vi "Set Target Velocity MM.vi"(9 "PointStreams":T3, 10 "Input (ft/s)":cluster{"LF":dbl, "LB":dbl, "RF":dbl, "RB":dbl}, 11 "Swerve motors":cluster{"LF":T6, "LB":T6, "RF":T6, "RB":T6}) -> (0 "error out":errorcluster, 3 "PointStreams Out":T2)   [LabVIEW 2020]
uses:
  <vilib>/Rock Robotics/WPI/MotorControl/WPI_MotorControlDeviceRef.ctl
  <vilib>/Rock Robotics/WPI/MotorControl/WPI_MotorControlType.ctl
  <vilib>/Rock Robotics/SystemInterfaces/DIO/FPGA_DIOPWMChannel.ctl
  <vilib>/Rock Robotics/WPI/PWM/WPI_PWMDeadband.ctl
  <vilib>/Rock Robotics/SystemInterfaces/DIO/FPGA_DIOChannel.ctl
  <vilib>/Rock Robotics/WPI/ThirdParty/Phoenix-LabVIEW/Motor Controller/Controls/CTRE_Phoenix_MotorControl_BufferedTrajectoryPointStream_DeviceRef.ctl
  <vilib>/Rock Robotics/WPI/ThirdParty/Phoenix-LabVIEW/Motor Controller/Controls/CTRE_Phoenix_MotorControl_MotionProfileTrajectoryPoint.ctl
  6b64e063-40b4-435e-b595-c1611d5f6bb1.vi
  <vilib>/Rock Robotics/WPI/ThirdParty/Phoenix-LabVIEW/Motor Controller/Get/CTRE_Phoenix_MotorController_GetSelectedSensorData.vi
  Framework/Robot Global Data.vi
  <vilib>/Rock Robotics/WPI/ThirdParty/Phoenix-LabVIEW/Motor Controller/Closed Loop/Motion Profile/CTRE_Phoenix_MotorControl_BufferedTrajectoryPointStream_WriteOne.vi
  <vilib>/ptbypt/NI_PtbyPt.lvlib
panel:
  out "integral x(t) 2":dbl format="%0.2f"
  out "integral x(t)":dbl format="%0.2f"
  in  "Current Pod":T4(ring)
  in  "Push PID":bool
  in  "Debug Mode":bool
  out "Drive Setpoints":T5(graph)
  in  "F":dbl
  in  "D":dbl
  in  "I":dbl
  in  "P":dbl
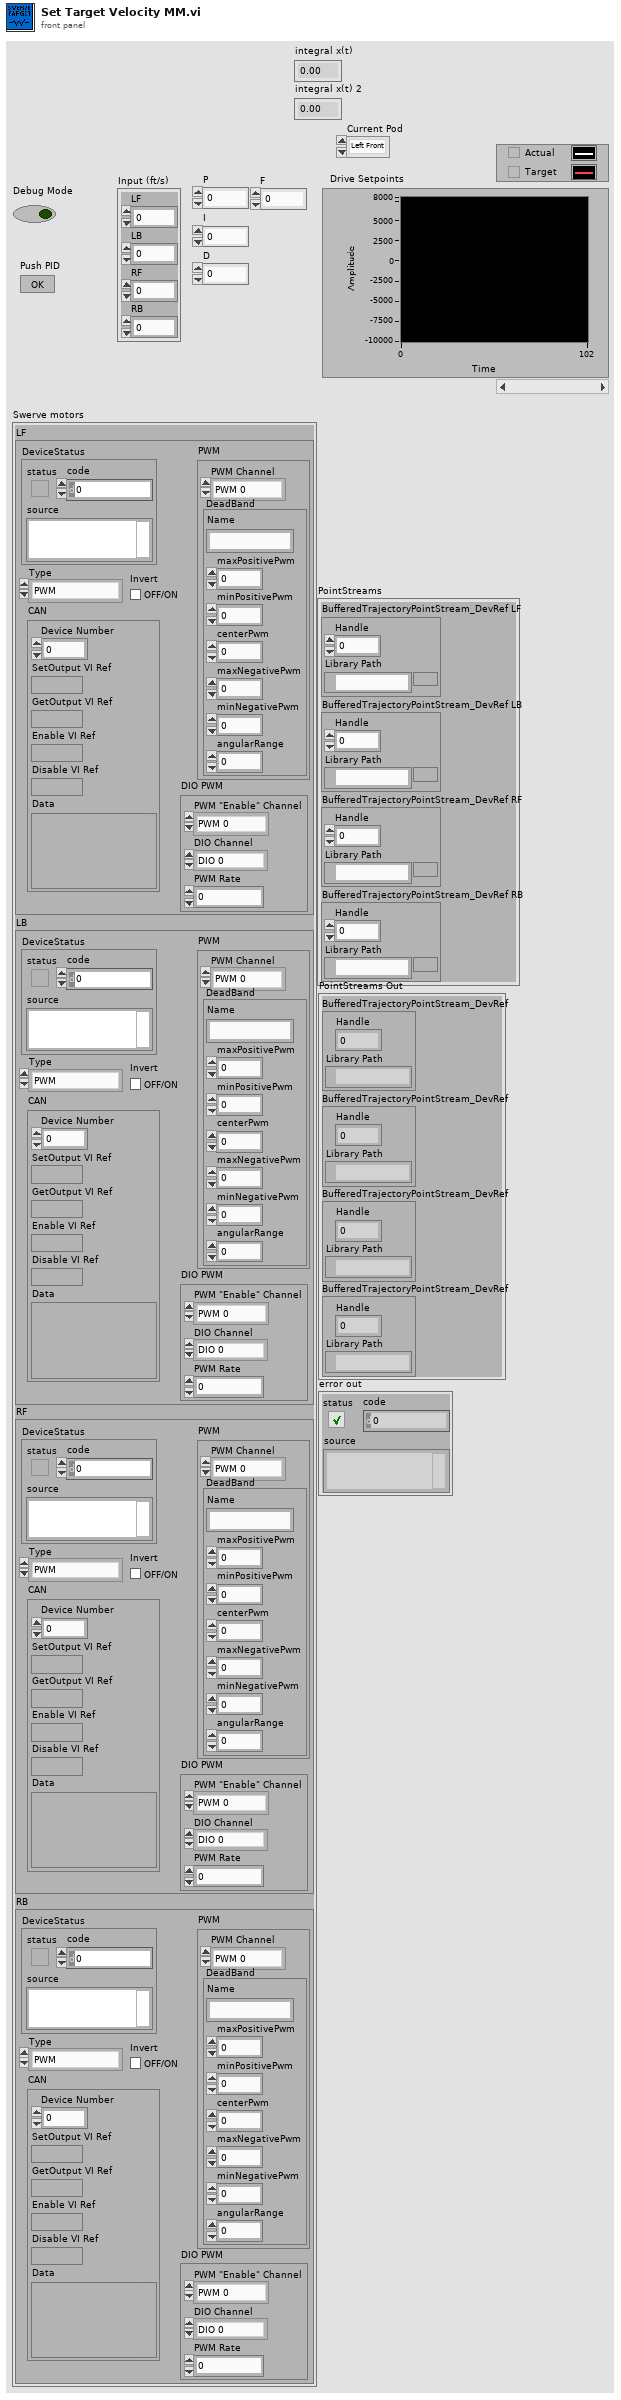
[diagram p1: front panel]
types:
  T1 = typedef "CTRE_Phoenix_MotorControl_BufferedTrajectoryPointStream_DeviceRef.ctl" = cluster{"Handle":u64, "Library Path":path}
  T2 = cluster{"BufferedTrajectoryPointStream_DevRef":T1, "BufferedTrajectoryPointStream_DevRef":T1, "BufferedTrajectoryPointStream_DevRef":T1, "BufferedTrajectoryPointStream_DevRef":T1}
  T3 = cluster{"BufferedTrajectoryPointStream_DevRef LF":T1, "BufferedTrajectoryPointStream_DevRef LB":T1, "BufferedTrajectoryPointStream_DevRef RF":T1, "BufferedTrajectoryPointStream_DevRef RB":T1}
  T4 = enum16{"Left Front", "Left Back", "Right Front", "Right Back"}
  T5 = cluster{"Velocity (Raw Sensor Units per 100 ms)":i32, "Velocity (ticks/ds)":dbl}
  T6 = typedef "WPI_MotorControlDeviceRef.ctl" = cluster{"DeviceStatus":errorcluster, "Type":T7, "PWM":cluster{"PWM Channel":T8, "DeadBand":T9}, "CAN":cluster{"Device Number":u8, "SetOutput VI Ref":variant, "GetOutput VI Ref":variant, "Enable VI Ref":variant, "Disable VI Ref":variant, "Data":variant}, "Invert":bool, "DIO PWM":cluster{"PWM \"Enable\" Channel":T8, "DIOChannel":T10, "PWM Rate":dbl}}
  T7 = typedef "WPI_MotorControlType.ctl" = enum16{"PWM", "CAN", "DIO PWM"}
  T8 = typedef "FPGA_DIOPWMChannel.ctl" = enum8{"PWM 0", "PWM 1", "PWM 2", "PWM 3", "PWM 4", "PWM 5", "PWM 6", "PWM 7", "PWM 8", "PWM 9", "PWM MXP 0", "PWM MXP 1", "PWM MXP 2", "PWM MXP 3", "PWM MXP 4", "PWM MXP 5", "PWM MXP 6", "PWM MXP 7", "PWM MXP 8", "PWM MXP 9", "Invalid"}
  T9 = typedef "WPI_PWMDeadband.ctl" = cluster{"Name":string, "maxPositivePwm":i32, "minPositivePwm":i32, "centerPwm":i32, "maxNegativePwm":i32, "minNegativePwm":i32, "angularRange":u16}
  T10 = typedef "FPGA_DIOChannel.ctl" = enum8{"DIO 0", "DIO 1", "DIO 2", "DIO 3", "DIO 4", "DIO 5", "DIO 6", "DIO 7", "DIO 8", "DIO 9", "DIO MXP 0", "DIO MXP 1", "DIO MXP 2", "DIO MXP 3", "DIO MXP 4", "DIO MXP 5", "DIO MXP 6", "DIO MXP 7", "DIO MXP 8", "DIO MXP 9", "DIO MXP 10", "DIO MXP 11", "DIO MXP 12", "DIO MXP 13", "DIO MXP 14", "DIO MXP 15", "SPI Port CS1", "SPI Port CS2", "SPI Port CS3", "SPI Port MISO", "SPI Port MOSI", "Invalid"}
  T11 = typedef "CTRE_Phoenix_MotorControl_MotionProfileTrajectoryPoint.ctl" = cluster{"Position":dbl, "Velocity":dbl, "Arbitrary Feed Forward":dbl, "Auxiliary Position":dbl, "Auxiliary Velocity":dbl, "Auxiliary Arbitrary Feed Forward":dbl, "Profile Slot Select":i32, "Auxiliary Profile Slot Select":i32, "isLastPoint?":bool, "Zero Position?":bool, "durationMs":u32, "Use Aux PID?":bool}
  T12 = cluster{"LF":bool, "LB":bool, "RF":bool, "RB":bool}
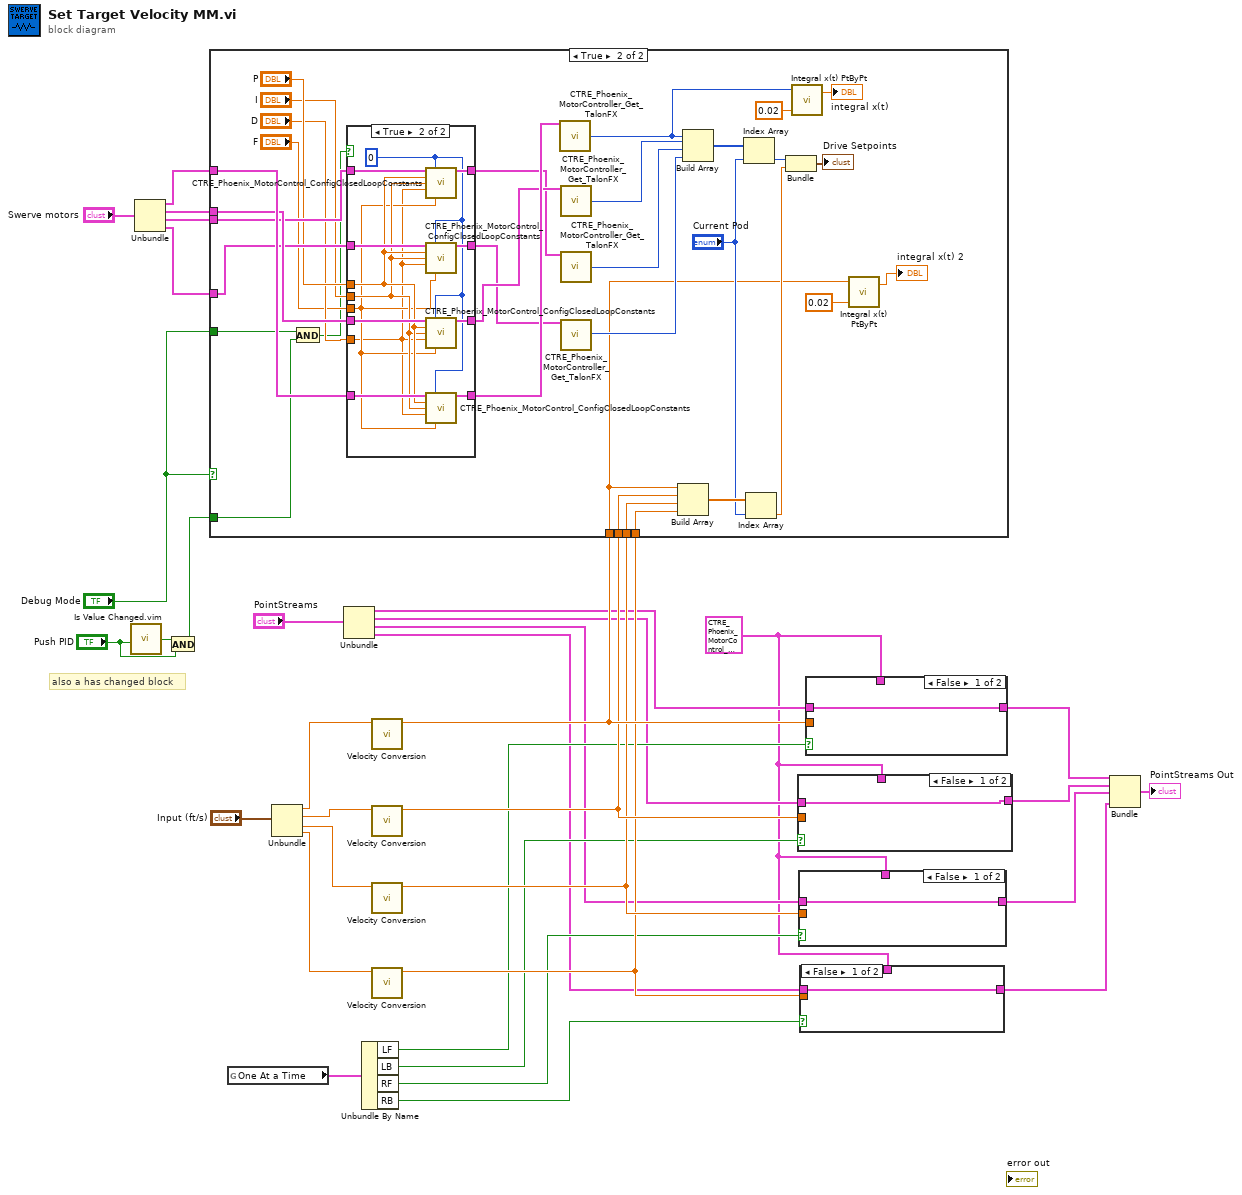
[diagram p0: block diagram]
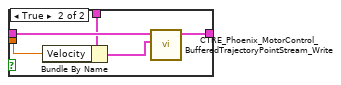
[diagram p2: hidden frame]
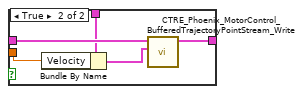
[diagram p3: hidden frame]
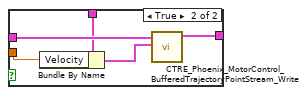
[diagram p4: hidden frame]
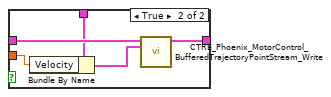
[diagram p5: hidden frame]
diagram:
  w6 = T11 {"Position"=0.0, "Velocity"=0.0, "Arbitrary Feed Forward"=0.0, "Auxiliary Position"=0.0, "Auxiliary Velocity"=0.0, "Auxiliary Arbitrary Feed Forward"=0.0, "Profile Slot Select"=0, "Auxiliary Profile Slot Select"=0, "isLastPoint?"=FALSE, "Zero Position?"=FALSE, "durationMs"=0, "Use Aux PID?"=FALSE} ("element")
  # "also a has changed block"
  n1 = call "Is Value Changed.vim"("value"="Push PID") -> ("changed or first call?"=w18:bool)
  n2 = Unbundle("Swerve motors") -> ("LF"=w33:T6, "LB"=w32:T6, "RF"=w31:T6, "RB"=w30:T6)
  n3 = And(x=w18, y="Push PID") -> (x .and. y?=w19:bool)
  n4 = global read "Robot Global Data.vi" "One At a Time"() -> (w16:T12)
  n5 = Unbundle("Input (ft/s)") -> ("LF"=w28:dbl, "LB"=w27:dbl, "RF"=w26:dbl, "RB"=w25:dbl)
  n6 = Unbundle("PointStreams") -> ("BufferedTrajectoryPointStream_DevRef LF"=w10:T1, "BufferedTrajectoryPointStream_DevRef LB"=w9:T1, "BufferedTrajectoryPointStream_DevRef RF"=w8:T1, "BufferedTrajectoryPointStream_DevRef RB"=w7:T1)
  n7 = Unbundle By Name(w16) -> ("LF"=w15:bool, "LB"=w14:bool, "RF"=w13:bool, "RB"=w12:bool)
  n8 = call "Velocity Conversion.vi"("Velocity (ft/s)"=w28) -> ("Velocity (ticks/ds)"=w24:dbl)  [unwired: 10 in]
  n9 = call "Velocity Conversion.vi"("Velocity (ft/s)"=w27) -> ("Velocity (ticks/ds)"=w23:dbl)  [unwired: 10 in]
  n10 = call "Velocity Conversion.vi"("Velocity (ft/s)"=w26) -> ("Velocity (ticks/ds)"=w22:dbl)  [unwired: 10 in]
  n11 = call "Velocity Conversion.vi"("Velocity (ft/s)"=w25) -> ("Velocity (ticks/ds)"=w21:dbl)  [unwired: 10 in]
  n12 = case shown="True" "Debug Mode" {
    tunnel: w33 -> [_ w67]
    tunnel: w32 -> [_ w66]
    tunnel: w31 -> [_ w65]
    tunnel: w30 -> [_ w64]
    tunnel: w24 -> [_ w36]
    tunnel: w23 -> [_ w49]
    tunnel: w22 -> [_ w48]
    tunnel: w21 -> [_ w47]
    tunnel: "Debug Mode" -> [_ w54]
    tunnel: w19 -> [_ w53]
    frame False {
    }
    frame True {
      n13 = And(x=w54, y=w53) -> (x .and. y?=w55:bool)
      n14 = case shown="True" w55 {
        tunnel: w67 -> [w71 w84]
        tunnel: w66 -> [w70 w83]
        tunnel: w65 -> [w69 w82]
        tunnel: w64 -> [w68 w81]
        tunnel: "P" -> [_ w80]
        tunnel: "I" -> [_ w79]
        tunnel: "D" -> [_ w72]
        tunnel: "F" -> [_ w78]
        tunnel: [w71 w77] -> w59
        tunnel: [w70 w76] -> w58
        tunnel: [w69 w75] -> w57
        tunnel: [w68 w74] -> w56
        frame False {
        }
        frame True {
          w73 = 0 ("slotIdx")
          n15 = call <vilib>:"CTRE_Phoenix_MotorControl_ConfigClosedLoopConstants.vi"("PhoenixMotorControlDevRef"=w82, "slotIdx"=w73, "P"=w80, "I"=w79, "D"=w72, "F"=w78) -> ("PhoenixMotorControlDevRef"=w75:T6)  [unwired: 8 in, 1 out]
          n16 = call <vilib>:"CTRE_Phoenix_MotorControl_ConfigClosedLoopConstants.vi"("PhoenixMotorControlDevRef"=w81, "slotIdx"=w73, "P"=w80, "I"=w79, "D"=w72, "F"=w78) -> ("PhoenixMotorControlDevRef"=w74:T6)  [unwired: 8 in, 1 out]
          n17 = call <vilib>:"CTRE_Phoenix_MotorControl_ConfigClosedLoopConstants.vi"("PhoenixMotorControlDevRef"=w83, "slotIdx"=w73, "P"=w80, "I"=w79, "D"=w72, "F"=w78) -> ("PhoenixMotorControlDevRef"=w76:T6)  [unwired: 8 in, 1 out]
          n18 = call <vilib>:"CTRE_Phoenix_MotorControl_ConfigClosedLoopConstants.vi"("PhoenixMotorControlDevRef"=w84, "slotIdx"=w73, "P"=w80, "I"=w79, "D"=w72, "F"=w78) -> ("PhoenixMotorControlDevRef"=w77:T6)  [unwired: 8 in, 1 out]
        }
      }
      n19 = call-poly <vilib>:"CTRE_Phoenix_MotorController_Get_TalonFX.vi"("PhoenixMotorControlDevRef"=w59) -> ("Velocity (Raw Sensor Units per 100 ms)"=w40:i32)  [unwired: 11 in, 3 out]
      n20 = call-poly <vilib>:"CTRE_Phoenix_MotorController_Get_TalonFX.vi"("PhoenixMotorControlDevRef"=w58) -> ("Velocity (Raw Sensor Units per 100 ms)"=w52:i32)  [unwired: 11 in, 3 out]
      n21 = call-poly <vilib>:"CTRE_Phoenix_MotorController_Get_TalonFX.vi"("PhoenixMotorControlDevRef"=w57) -> ("Velocity (Raw Sensor Units per 100 ms)"=w51:i32)  [unwired: 11 in, 3 out]
      n22 = call-poly <vilib>:"CTRE_Phoenix_MotorController_Get_TalonFX.vi"("PhoenixMotorControlDevRef"=w56) -> ("Velocity (Raw Sensor Units per 100 ms)"=w50:i32)  [unwired: 11 in, 3 out]
      n23 = Build Array(w36, w49, w48, w47) -> (w45:dbl[])
      n24 = Build Array(w40, w52, w51, w50) -> (w46:i32[])
      n25 = Index Array(array=w46, index="Current Pod") -> (element=w43:i32)
      n26 = Index Array(array=w45, index="Current Pod") -> (element=w42:dbl)
      n27 = Bundle("Velocity (Raw Sensor Units per 100 ms)"=w43, "Velocity (ticks/ds)"=w42) -> (→"Drive Setpoints":T5)  [unwired: 1 in]
      n28 = call <vilib>:"Integral x(t) PtByPt.vi"("dt"=0.02, "x"=w40) -> ("integral x(t)"=→"integral x(t)":dbl)  [unwired: 2 in, 1 out]
      n29 = call <vilib>:"Integral x(t) PtByPt.vi"("dt"=0.02, "x"=w36) -> ("integral x(t)"=→"integral x(t) 2":dbl)  [unwired: 2 in, 1 out]
    }
  }
  n30 = case shown="False" w14 {
    tunnel: w23 -> [_ w89]
    tunnel: w9 -> [w85 w90]
    tunnel: w6 -> [_ w87]
    tunnel: [w85 w86] -> w4
    frame False {
    }
    frame True {
      n31 = Bundle By Name(cluster=w87, "Velocity"=w89) -> (w88:T11)
      n32 = call-poly <vilib>:"CTRE_Phoenix_MotorControl_BufferedTrajectoryPointStream_Write.vi"("Trajectory Point"=w88, "BufferedTrajectoryPointStream_DevRef"=w90) -> ("BufferedTrajectoryPointStream_DevRef"=w86:T1)  [unwired: 8 in, 1 out]
    }
  }
  n33 = case shown="False" w13 {
    tunnel: w22 -> [_ w95]
    tunnel: w8 -> [w91 w96]
    tunnel: w6 -> [_ w94]
    tunnel: [w91 w92] -> w3
    frame False {
    }
    frame True {
      n34 = Bundle By Name(cluster=w94, "Velocity"=w95) -> (w93:T11)
      n35 = call-poly <vilib>:"CTRE_Phoenix_MotorControl_BufferedTrajectoryPointStream_Write.vi"("Trajectory Point"=w93, "BufferedTrajectoryPointStream_DevRef"=w96) -> ("BufferedTrajectoryPointStream_DevRef"=w92:T1)  [unwired: 8 in, 1 out]
    }
  }
  n36 = case shown="False" w12 {
    tunnel: w21 -> [_ w101]
    tunnel: w7 -> [w97 w102]
    tunnel: w6 -> [_ w100]
    tunnel: [w97 w98] -> w2
    frame False {
    }
    frame True {
      n37 = Bundle By Name(cluster=w100, "Velocity"=w101) -> (w99:T11)
      n38 = call-poly <vilib>:"CTRE_Phoenix_MotorControl_BufferedTrajectoryPointStream_Write.vi"("Trajectory Point"=w99, "BufferedTrajectoryPointStream_DevRef"=w102) -> ("BufferedTrajectoryPointStream_DevRef"=w98:T1)  [unwired: 8 in, 1 out]
    }
  }
  n39 = case shown="False" w15 {
    tunnel: w24 -> [_ w105]
    tunnel: w10 -> [w103 w108]
    tunnel: w6 -> [_ w107]
    tunnel: [w103 w104] -> w5
    frame False {
    }
    frame True {
      n40 = Bundle By Name(cluster=w107, "Velocity"=w105) -> (w106:T11)
      n41 = call-poly <vilib>:"CTRE_Phoenix_MotorControl_BufferedTrajectoryPointStream_Write.vi"("Trajectory Point"=w106, "BufferedTrajectoryPointStream_DevRef"=w108) -> ("BufferedTrajectoryPointStream_DevRef"=w104:T1)  [unwired: 8 in, 1 out]
    }
  }
  n42 = Bundle("BufferedTrajectoryPointStream_DevRef"=w5, "BufferedTrajectoryPointStream_DevRef"=w4, "BufferedTrajectoryPointStream_DevRef"=w3, "BufferedTrajectoryPointStream_DevRef"=w2) -> (→"PointStreams Out":T2)  [unwired: 1 in]
